vi "Instrument Base_Create.vi"(8 "Error In":errorcluster, 10 "IConfigure":refnum<class "IConfigure.lvclass">, 11 "reference in":refnum<class "Instr Base.lvclass">) -> (0 "Error Out":errorcluster, 3 "reference out":refnum<class "Instr Base.lvclass">)   [LabVIEW 2023, in "HAL GOOP4.lvlib" / "Instr Base.lvclass"]
uses:
  Instr Base.lvclass
  Interfaces/IConfigure/IConfigure.lvclass
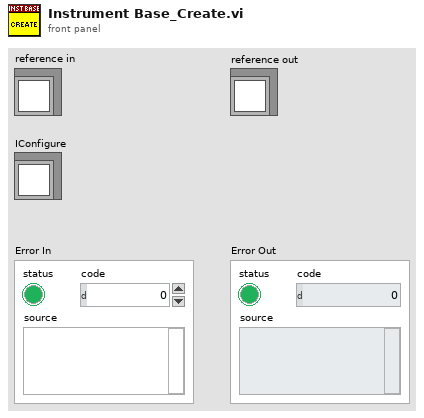
[diagram p1: front panel]
types:
  T1 = typedef "HAL GOOP4.lvlib/Instrument Base.lvclass/ObjectAttributes.ctl" = cluster{"IConfigure":refnum<class "IConfigure.lvclass">, "Ref Count":u8}
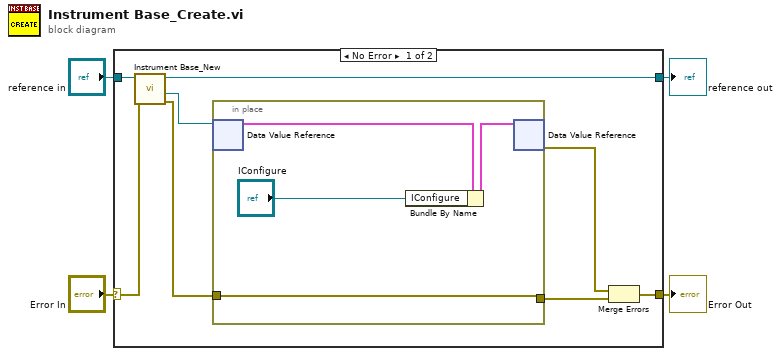
[diagram p0: block diagram]
diagram:
  n1 = case shown="No Error" "Error In" {
    selector: "Error In" -> [w11 w18]
    tunnel: [w9 w18] -> w3
    tunnel: "reference in" -> [w12 w17]
    tunnel: [w6 w17] -> w1
    frame No Error {
      n2 = call "Instrument Base_New.vi"("Error In"=w11, "reference in"=w12) -> ("Error Out"=w5:errorcluster, "DVRRefOut"=w8:refnum<data-value>, "reference out"=w6:refnum<class "Instr Base.lvclass">)  [unwired: 6 in, 1 out]
      n3 = in-place {
        in-place-border: [w14] -> w10
        in-place-border: w5 -> [w14]
        n4 = in-place-dvr #1(w8) -> (w16:T1)  [unwired: 1 out]
        n5 = Bundle By Name(cluster=w16, "IConfigure"="IConfigure") -> (w15:T1)
        n6 = in-place-dvr #1(w15) -> (w7:errorcluster)  [unwired: 1 out]
      }
      n7 = Merge Errors(w7, w10) -> (w9:errorcluster)
    }
    frame Error {
      # "VI-TechBaseTemplate_Simple_4x4x4"
    }
  }
  "Error Out" <- w3
  "reference out" <- w1
